vi "Project 6 Help.vi"() -> (0 "Velocity v(t)":cluster{"X":dbl[], "Y":dbl[]}[](graph) caption="XY Graph", 1 "Pos x(t)":cluster{"X":dbl[], "Y":dbl[]}[](graph) caption="XY Graph", 5 "error out 2":errorcluster caption="error out")   [LabVIEW 2019]
uses:
  <vilib>/Analysis/3filter.llb/Filter Passband Type.ctl
  <vilib>/Analysis/baseanly.llb/Mean (DBL).vi
  <vilib>/Analysis/3filter.llb/Butterworth Filter (DBL).vi
  <vilib>/imath/engines/lvmath2/RunTimeEngine/Managers/WorkSpace/UID Generator.vi
  <vilib>/imath/engines/lvmath2/RunTimeEngine/RunTimeType/NIMS_RunTimeType_From StrictType (excl LVString).vi
  <instcachedir>/0/NIMS_RunTimeType_From StrictType (excl LVString)_D8AFBA86A94845AAA577C895450664BD.lvgen/NIMS_RunTimeType_From StrictType (excl LVString)_D8AFBA86A94845AAA577C895450664BD_000.vi
  <vilib>/imath/engines/lvmath2/RunTimeEngine/LocalVariableDefStatement/MC_LocalVariableDefStatement_Display.vi
  <vilib>/imath/engines/lvmath2/RunTimeEngine/BuiltInFunctions/sin/NIMS_sin(C).vi
  <instcachedir>/0/NIMS_sin(C)_6504C6AC704B4661870B0E93397B11C4.lvgen/NIMS_sin(C)_6504C6AC704B4661870B0E93397B11C4_001.vi
  <vilib>/imath/engines/lvmath2/RunTimeEngine/BuiltInFunctions/cos/NIMS_cos(C).vi
  <instcachedir>/0/NIMS_cos(C)_BED070B05FDB4939A63CB05E18805866.lvgen/NIMS_cos(C)_BED070B05FDB4939A63CB05E18805866_001.vi
  <vilib>/imath/engines/lvmath2/RunTimeEngine/Managers/SymbolTable/Clear UID.vi
  <vilib>/imath/engines/lvmath2/RunTimeEngine/NodeEndStatement/NIMS_NodeEndStatement_Output.vi
  <instcachedir>/0/NIMS_NodeEndStatement_Output_53EC0D466D134D7ABD903AC30B43404B.lvgen/NIMS_NodeEndStatement_Output_53EC0D466D134D7ABD903AC30B43404B_000.vi
  <instcachedir>/0/NIMS_NodeEndStatement_Output_53EC0D466D134D7ABD903AC30B43404B.lvgen/NIMS_NodeEndStatement_Output_53EC0D466D134D7ABD903AC30B43404B_005.vi
  <vilib>/imath/engines/lvmath2/RunTimeEngine/ErrorHandling/NIMS_Finalize Error.vi
  <vilib>/Analysis/NI_AAL_SigProc.lvlib
  <vilib>/Analysis/NI_AALPro.lvlib
  <vilib>/Analysis/NI_AALBase.lvlib
  <vilib>/imath/engines/lvmath2/RunTimeEngine/Managers/SymbolTable/NIMS_WorkSpace.lvlib
panel:
  out "Waveform Graph":dbl[](graph)
  out "XY Graph":cluster{"X":dbl[], "Y":dbl[]}[](graph)
  out "Amplitude":dbl
  out "damping":dbl
  out "raw data":dbl[](array[numeric])
  out "time array":dbl[](array[numeric])
  out "dt":dbl
  out "Omega":dbl
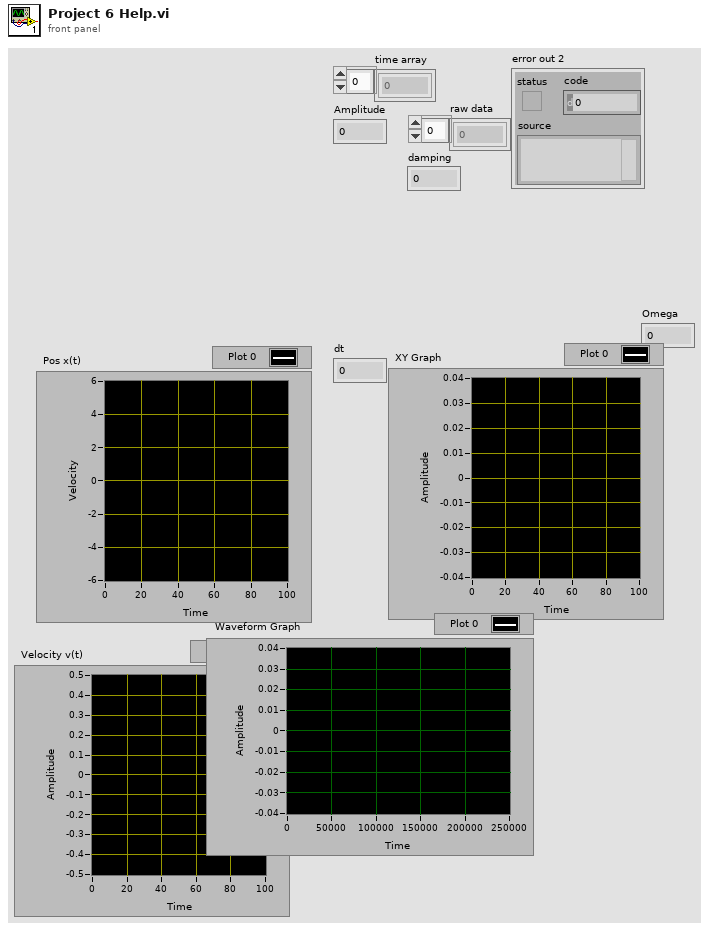
[diagram p1: front panel]
types:
  T1 = typedef "NI_AALBase.lvlib/Filter Passband Type.ctl" = enum32{"Lowpass", "Highpass", "Bandpass", "Bandstop"}
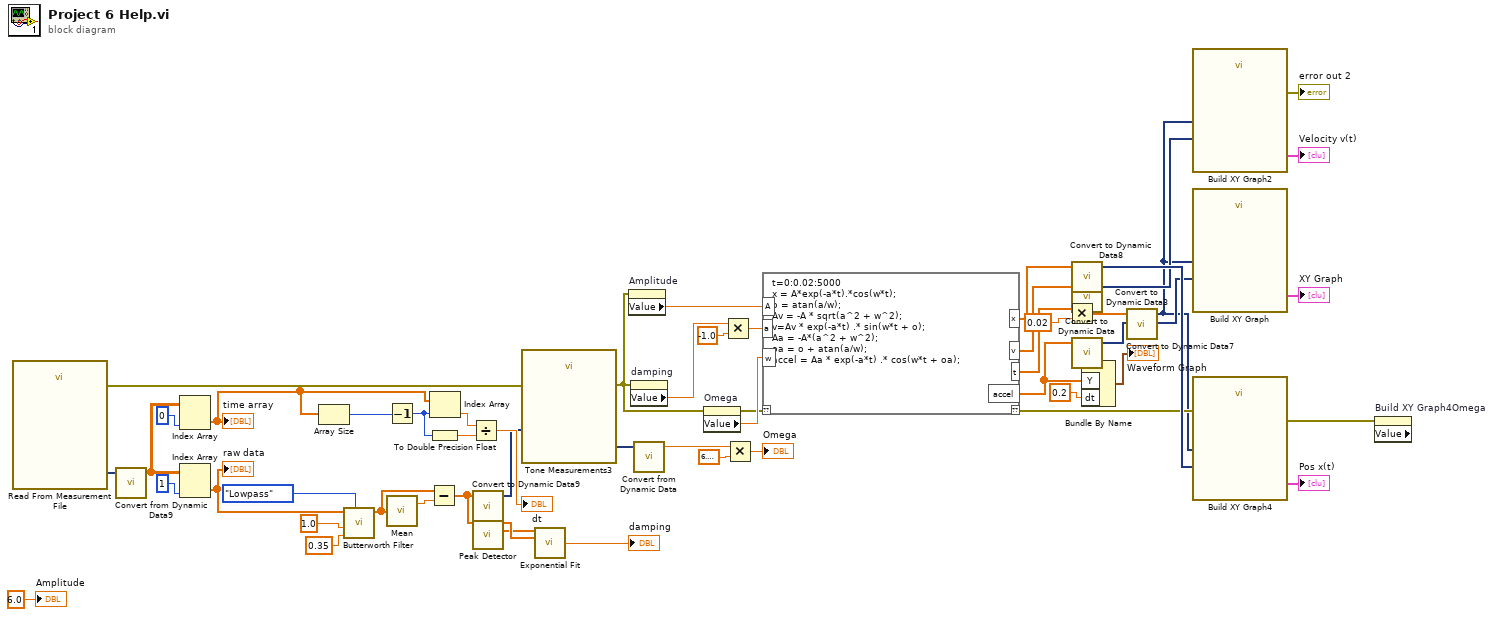
[diagram p0: block diagram]
diagram:
  n1 = call "Read From Measurement File"() -> ("error out"=w18:errorcluster, "Signals"=w34:dynamicdata)  [unwired: 6 in, 4 out]
  n2 = call "Convert from Dynamic Data9"("Dynamic Data Type"=w34) -> ("Array"=w44:dbl[][])  [unwired: 3 in]
  n3 = Index Array(array=w44, index (col)=0 ("disabled index (col)")) -> (element=w38:dbl[])  [unwired: 1 in]
  "time array" <- w38
  n4 = Index Array(array=w44, index (col)=1 ("disabled index (col)")) -> (element=w30:dbl[])  [unwired: 1 in]
  "raw data" <- w30
  n5 = Array Size(array=w38) -> (size(s)=w42:i32)
  n6 = call-poly <vilib>:"Butterworth Filter.vi"("filter type"=Filter_Passband_Type."Lowpass", "low cutoff freq: fl"=0.35, "high cutoff freq: fh"=1.0, "X"=w30) -> ("Filtered X"=w29:dbl[])  [unwired: 4 in, 1 out]
  n7 = Decrement(x=w42) -> (x-1=w40:i32)
  n8 = call-poly <vilib>:"Mean.vi"("X"=w29) -> ("mean"=w28:dbl)  [unwired: 1 out]
  n9 = Subtract(x=w29, y=w28) -> (x-y=w26:dbl[])
  n10 = Index Array(array=w38, index=w40) -> (element=w41:dbl)
  n11 = To Double Precision Float(number=w40) -> (double precision float=w39:dbl)
  n12 = Divide(x=w41, y=w39) -> (x/y=→"dt":dbl)
  n13 = call "Convert to Dynamic Data9"("Array"=w26) -> ("Dynamic Data Type"=w27:dynamicdata)  [unwired: 3 in]
  n14 = call <vilib>:"Peak Detector.vi"("X"=w26) -> ("Amplitudes"=w24:dbl[], "Locations"=w25:dbl[])  [unwired: 6 in, 3 out]
  n15 = call "Tone Measurements3"("error in (no error)"=w18, "Signals"=w27) -> ("error out"=w14:errorcluster, "Frequency"=w22:dynamicdata)  [unwired: 7 in, 1 out]
  n16 = call <vilib>:"Exponential Fit.vi"("Y"=w24, "X"=w25) -> ("damping"=→"damping":dbl)  [unwired: 8 in, 5 out]
  n17 = property on="Amplitude" class="DigNum (strict)"(error in=w14) -> ("Value"=w15:dbl)  [unwired: 1 in, 2 out]
  n18 = property on="damping" class="DigNum (strict)"(error in=w14) -> ("Value"=w20:dbl)  [unwired: 1 in, 2 out]
  n19 = call "Convert from Dynamic Data"("Dynamic Data Type"=w22) -> ("Scalar"=w21:dbl)  [unwired: 3 in]
  n20 = property on="Omega" class="DigNum (strict)"(error in=w14) -> (error out=w12:errorcluster, "Value"=w19:dbl)  [unwired: 1 in, 1 out]
  n21 = Multiply(x=w20, y=-1.0) -> (x*y=w10:dbl)
  n22 = Multiply(x=w21, y=6.283185307179586) -> (x*y=→"Omega":dbl)
  n23 = mathscript code="t=0:0.02:5000\nx = A*exp(-a*t).*cos(w*t);\no = atan(a/w);\nAv = -A * sqrt(a^2 + w^2);\nv=Av * exp(-a*t) .* sin(w*t + o);\nAa = -A*(a^2 + w^2);\noa = o + atan(a/w);\naccel = Aa * exp(-a*t) .* cos(w*t + oa);"("??"=w12, "A"=w15, "a"=w10, "w"=w19) -> ("??"=w17:errorcluster, "x"=w35:dbl[], "v"=w13:cdb[], "t"=w11:dbl[], "accel"=w5:cdb[])
  n24 = Multiply(x=w11, y=0.02) -> (x*y=w2:dbl[])
  n25 = call "Convert to Dynamic Data8"("Array"=w35) -> ("Dynamic Data Type"=w51:dynamicdata)  [unwired: 3 in]
  n26 = call "Convert to Dynamic Data3"("Array"=w13) -> ("Dynamic Data Type"=w47:dynamicdata)  [unwired: 3 in]
  n27 = call "Convert to Dynamic Data"("Array"=w5) -> ("Dynamic Data Type"=w8:dynamicdata)  [unwired: 3 in]
  n28 = Bundle By Name("Y"=w5, "dt"=0.2) -> (→"Waveform Graph":waveform(cdb))  [unwired: 1 in]
  n29 = call "Convert to Dynamic Data7"("Array"=w2) -> ("Dynamic Data Type"=w7:dynamicdata)  [unwired: 3 in]
  n30 = call "Build XY Graph2"("Y Input"=w47, "X Input"=w7) -> ("error out"=→"error out 2":errorcluster, "XY Graph"=→"Velocity v(t)":cluster{"X":dbl[], "Y":dbl[]}[])  [unwired: 8 in]
  n31 = call "Build XY Graph"("Y Input"=w8, "X Input"=w7) -> ("XY Graph"=→"XY Graph":cluster{"X":dbl[], "Y":dbl[]}[])  [unwired: 8 in, 1 out]
  n32 = call "Build XY Graph4"("error in (no error)"=w17, "Y Input"=w51, "X Input"=w7) -> ("error out"=w50:errorcluster, "XY Graph"=→"Pos x(t)":cluster{"X":dbl[], "Y":dbl[]}[])  [unwired: 7 in]
  n33 = property on="Build XY Graph4Omega" class="DigNum (strict)" props=["Value"](error in=w50) -> ()  [unwired: 1 in, 3 out]
  "Amplitude" <- 6.0
